vi "Set_Connection_Type.vi"(8 "error in (no error)":errorcluster caption="entrée d'erreur (pas d'erreur)", 10 "Connection_Type":string, 11 "Flash_Jlink en entrée":refnum<class "Flash_Jlink.lvclass">) -> (0 "error out":errorcluster caption="sortie d'erreur", 3 "Flash_Jlink en sortie":refnum<class "Flash_Jlink.lvclass">)   [LabVIEW 2020, in "Library Test.lvlib" / "Flash_Jlink.lvclass"]
uses:
  Flash_Jlink.lvclass
  Flash_Jlink.lvclass/Flash_Jlink.ctl
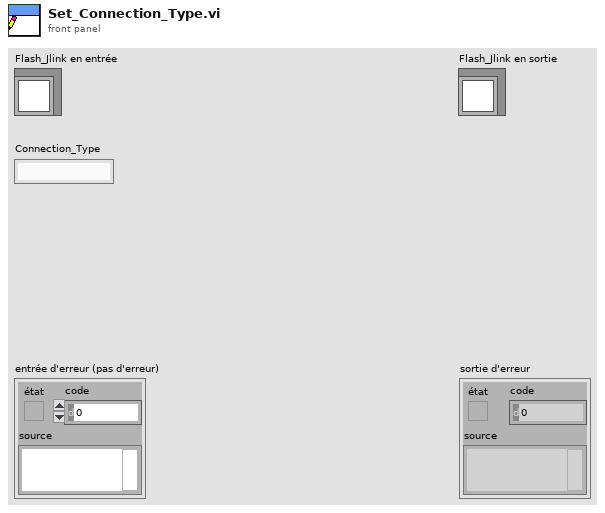
[diagram p1: front panel]
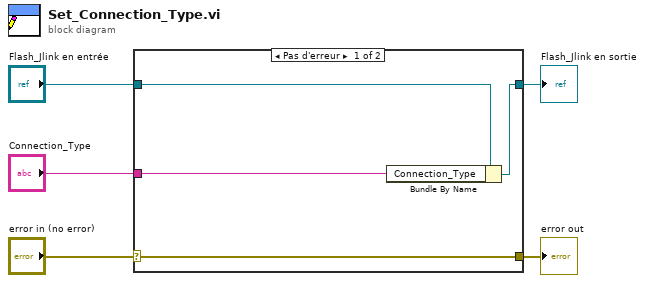
[diagram p0: block diagram]
diagram:
  n1 = case shown="Pas d'erreur" "error in (no error)" {
    selector: "error in (no error)" -> [w9 w10]
    tunnel: [w9 w10] -> w4
    tunnel: [w7 w11] -> w2
    tunnel: "Flash_Jlink en entrée" -> [w8 w11]
    tunnel: "Connection_Type" -> [w6 _]
    frame No Error {
      n2 = Bundle By Name(cluster=w8, "Connection_Type"=w6) -> (w7:refnum<class "Flash_Jlink.lvclass">)
    }
    frame Error {
    }
  }
  "error out" <- w4
  "Flash_Jlink en sortie" <- w2
